vi "next chunk - read-write freq PID file.vi"(4 "frequency":dbl, 6 "temperature":dbl, 7 "PID action":T1, 8 "freq PID file OUT":string="peak_PID_scratch.dat", 9 "freq PID file IN":string="peak_PID.dat", 11 "sweep folder path":path) -> (0 "temperatures":i32[](array[numeric]), 1 "frequencies":dbl[][](array[numeric]), 2 "PID freq":dbl[](array[numeric]), 3 "sweep folder path out":path)   [LabVIEW 2010]
uses:
  next chunk read-write PID -- action.ctl
  <vilib>/Utility/file.llb/Read From Spreadsheet File (string).vi
  <vilib>/Utility/file.llb/Write To Spreadsheet File (string).vi
panel:
  out "number":i32=9
  out "first line":string="Temperature(K)\tFrequency(kHz)\tGamma(kHz)\tDeltaFreq(kHz)\tTime(min)"
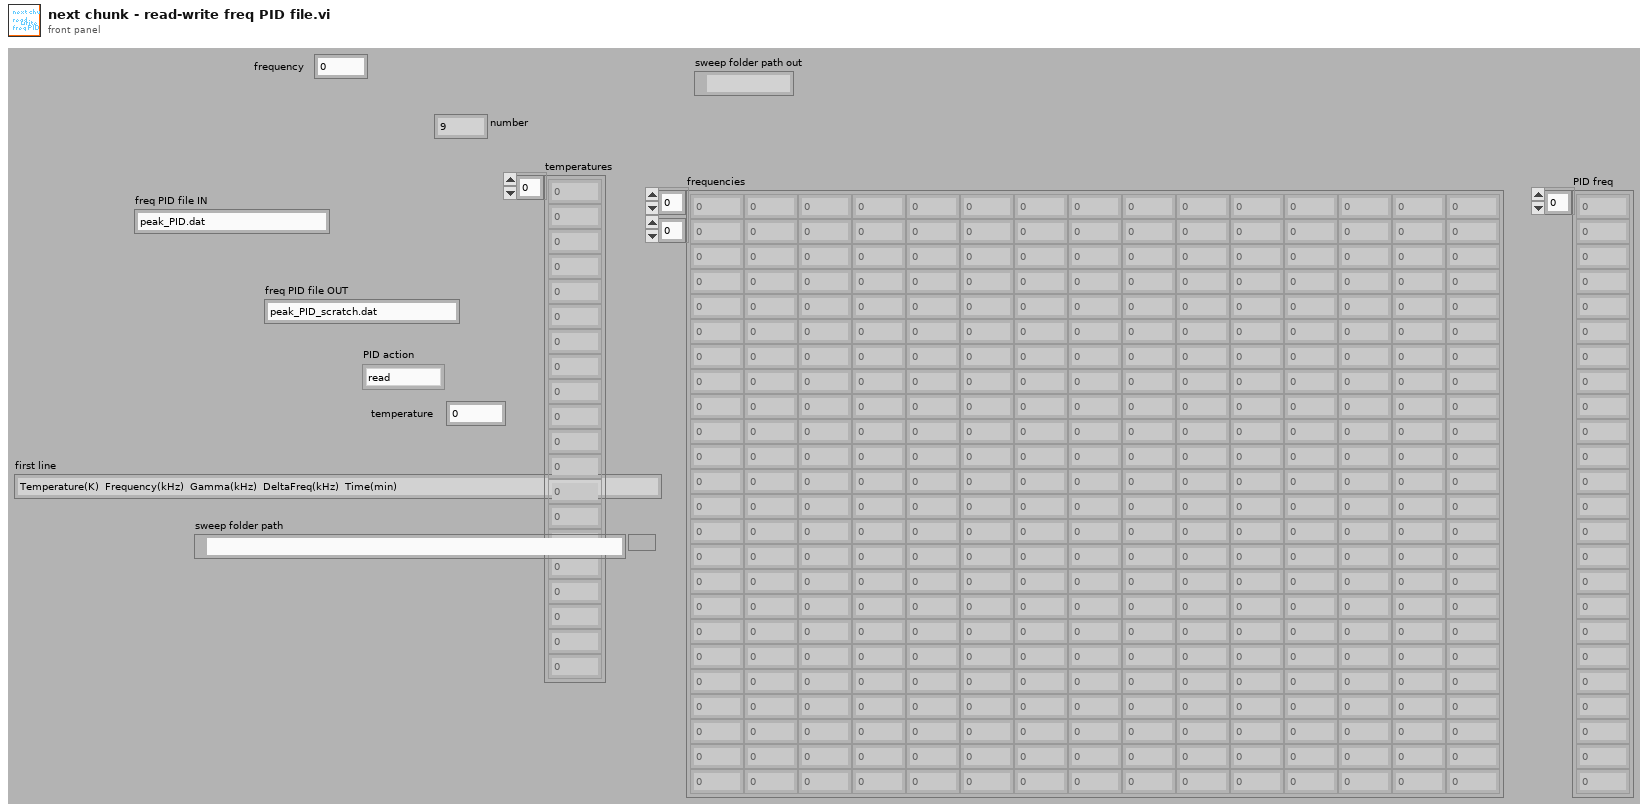
[diagram p1: front panel]
types:
  T1 = typedef "next chunk read-write PID -- action.ctl" = enum16{"read", "interpolate", "append", "write", ""}
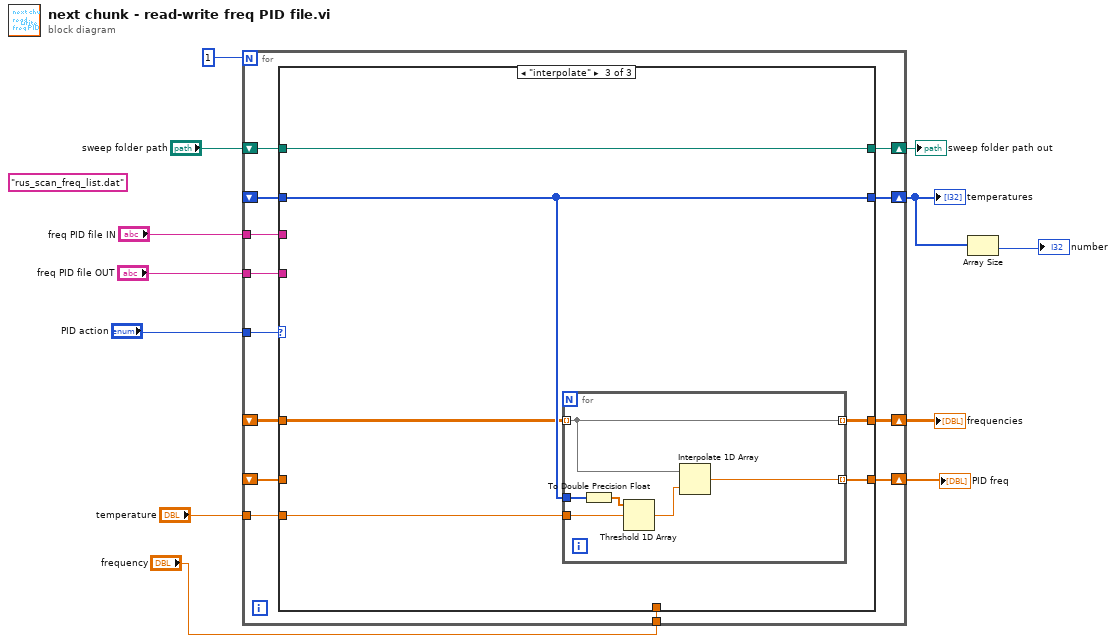
[diagram p0: block diagram]
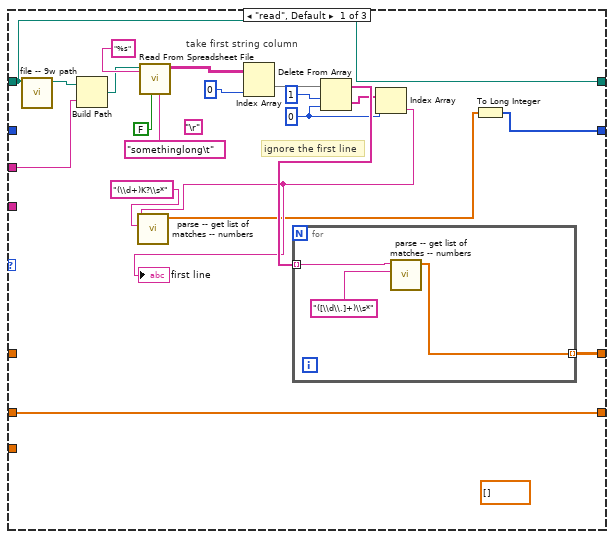
[diagram p2: hidden frame]
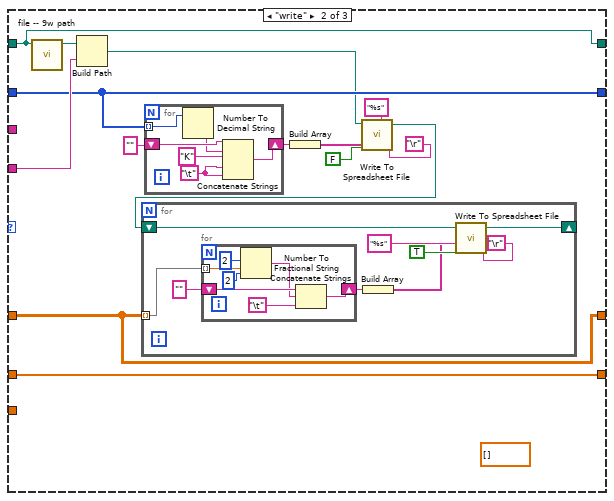
[diagram p3: hidden frame]
diagram:
  (unwired) "rus_scan_freq_list.dat" ("delimiter (\\t)")
  n1 = for {
    N: 1 -> [_]
    tunnel: "temperature" -> [w24]
    tunnel: "freq PID file IN" -> [w21]
    tunnel: "PID action" -> [w19]
    shift-right: [w25] -> w12
    shift-left: _ -> [w17]
    shift-right: [w20] -> w5
    shift-left: _ -> [w18]
    shift-right: [w23] -> w10
    shift-left: _ -> [w16]
    tunnel: "freq PID file OUT" -> [w15]
    tunnel: "frequency" -> [w14]
    shift-right: [w13] -> w1
    shift-left: "sweep folder path" -> [w22]
    n2 = case shown="\"interpolate\"" w19 {
      tunnel: [w35 w50 w90] -> w25
      tunnel: w24 -> [_ _ w89]
      tunnel: [w30 w61 w88] -> w23
      tunnel: w22 -> [w26 w49 w85]
      tunnel: w21 -> [w34 _ _]
      tunnel: [w28 w58 w87] -> w20
      tunnel: w18 -> [_ w58 w87]
      tunnel: w17 -> [_ w50 w86]
      tunnel: w16 -> [w30 w61 _]
      tunnel: w15 -> [_ w60 _]
      tunnel: w14 -> [_ _ _]
      tunnel: [w26 w49 w85] -> w13
      frame "read", Default {
        (unwired) dbl[] []
        w36 = 0 ("index")
        (unwired) "\r"
        # "take first string column"
        # "ignore the first line"
        n3 = call "file -- 9w path.vi"("sweep folder"=w26) -> ("9w path"=w27:path)  [unwired: 10 in]
        n4 = Build Path(base path=w27, name or relative path=w34) -> (appended path=w33:path)
        n5 = call-poly <vilib>:"Read From Spreadsheet File.vi"("delimiter (\\t)"="somethinglong\t" ("delimiter (\\t)"), "transpose (no:F)"=FALSE ("append to file? (new file:F)"), "format (%s)"="%s", "file path (dialog if empty)"=w33) -> ("all rows"=w42:string[][])  [unwired: 3 in, 4 out]
        n6 = Index Array(array=w42, index (col)=0 ("disabled index (col)")) -> (element=w40:string[])  [unwired: 1 in]
        n7 = Delete From Array(array=w40, length=1, index=w36) -> (deleted portion=w37:string[], array with subset deleted=w38:string[])
        n8 = for {
          tunnel: w38 -> [w48] mode=indexing
          tunnel: [w46] -> w35 mode=indexing
          n9 = call "parse -- get list of matches -- numbers.vi"("regexp"="([\\d\\.]+)\\s*", "string"=w48) -> ("Array of numbers"=w46:dbl[])  [unwired: 6 in, 3 out]
        }
        n10 = Index Array(array=w37, index=w36) -> (element=w32:string)
        "first line" <- w32
        n11 = call "parse -- get list of matches -- numbers.vi"("regexp"="(\\d+)K?\\s*", "string"=w32) -> ("Array of numbers"=w29:dbl[])  [unwired: 6 in, 3 out]
        n12 = To Long Integer(number=w29) -> (32bit integer=w28:i32[])
      }
      frame "write" {
        (unwired) dbl[] []
        n13 = call "file -- 9w path.vi"("sweep folder"=w49) -> ("9w path"=w62:path)  [unwired: 10 in]
        n14 = Build Path(base path=w62, name or relative path=w60) -> (appended path=w52:path)
        n15 = for {
          tunnel: w58 -> [w68] mode=indexing
          shift-right: [w66] -> w54
          shift-left: "" ("format (%s)") -> [w67]
          w64 = "\t"
          n16 = Number To Decimal String(number=w68) -> (decimal integer string=w65:string)  [unwired: 1 in]
          n17 = Concatenate Strings(w67, w65, "K" ("format (%s)"), w64, w64) -> (w66:string)
        }
        n18 = Build Array(w54) -> (w53:string[])
        n19 = call-poly <vilib>:"Write To Spreadsheet File.vi"("delimiter (\\t)"="\r", "format (%s)"="%s", "append to file? (new file:F)"=FALSE, "1D data"=w53, "file path (dialog if empty)"=w52) -> ("new file path (Not A Path if cancelled)"=w51:path)  [unwired: 3 in]
        n20 = for {
          tunnel: w50 -> [w70] mode=indexing
          shift-right: [w75] -> _
          shift-left: w51 -> [w76]
          n21 = for {
            tunnel: w70 -> [w84] mode=indexing
            shift-right: [w82] -> w71
            shift-left: "" ("format (%s)") -> [w83]
            n22 = Number To Fractional String(number=w84, width (-)=i16 2, precision (6)=i16 2 ("width (-)")) -> (F-format string=w81:string)  [unwired: 1 in]
            n23 = Concatenate Strings(w83, w81, "\t") -> (w82:string)
          }
          n24 = Build Array(w71) -> (w69:string[])
          n25 = call-poly <vilib>:"Write To Spreadsheet File.vi"("delimiter (\\t)"="\r", "format (%s)"="%s", "append to file? (new file:F)"=TRUE, "1D data"=w69, "file path (dialog if empty)"=w76) -> ("new file path (Not A Path if cancelled)"=w75:path)  [unwired: 3 in]
        }
      }
      frame "interpolate" {
        n26 = for {
          tunnel: [w94] -> w90 mode=indexing
          tunnel: w87 -> [w92]
          tunnel: w89 -> [w93]
          tunnel: [w95] -> w88 mode=indexing
          tunnel: w86 -> [w94] mode=indexing
          n27 = To Double Precision Float(number=w92) -> (double precision float=w91:dbl[])
          n28 = Threshold 1D Array(2:w93, 3:w91) -> (0:w96:dbl)  [unwired: 1 in]
          n29 = Interpolate 1D Array(1:w96, 2:w94) -> (0:w95:dbl)
        }
      }
    }
  }
  "frequencies" <- w12
  "temperatures" <- w5
  "PID freq" <- w10
  "sweep folder path out" <- w1
  n30 = Array Size(array=w5) -> (size(s)=→"number":i32)
